vi "PH_BlackBox.set modified data.vi"(0 "i ref in":refnum<vi>, 2 "i attribute":T1={"BB Remote Controlled?"=FALSE, "GUI Refs"={"MOVE IN"=refnum, "MOVE"=refnum, "IN"=refnum, "OUT"=refnum, "REMOTE"=refnum, "GUI-Knob Move"=refnum, "GUI-Knob Move in"=refnum, "POWER ON"=refnum, "Delete"=refnum, "Function Textfield"=refnum}, "Position IN"=0, "Position OUT"=0, "BB Remote Controlled by other Instance?"=FALSE, "Recipient"="N/A", "Number"=0, "Caption Move"="", "Caption Out"="", "Caption In"=""} {"Position OUT" items=["no info", "off/false/out", "on/true/in", "Failure", "Alarm", "Status 1", "Status 2", "Status 3"]; "Position IN" items=["no info", "off/false/out", "on/true/in", "Failure", "Alarm", "Status 1", "Status 2", "Status 3"]}, 5 "error in (no error)":errorcluster) -> (14 "i ref out":refnum<vi>, 19 "error out":errorcluster)   [LabVIEW 2014, in "PH_BlackBox.lvlib"]
doc: "Writes the data into the attribute of an object. Then, the attribute dara are unlocked using the \"release\" method. Prior to calling THIS method, the attribute data must have been locked using the methods \"lock\" or \"get data to modify\".\n\n\nLicense Agreement for this software:\n\nCopyright (C)\nGesellschaft für Schwerionenforschung, GSI\nPlanckstr. 1\n64291 Darmstadt\nGermany\n\nContact: D.Beck@gsi.de \n\nThis program is free software; you can redistribute it and/or modify it under the terms of the GNU General Public License as published by the Free Software Foundation; either version 2 of the license, or (at your option) any later version.\n\nThis program is distributed in the hope that it will be useful, but WITHOUT ANY WARRANTY; without even the implied warranty of MERCHANTABILITY or FITNESS FOR A PARTICULAR PURPOSE. See the GNU General License for more details (http://www.gnu.org).\n\nGesellschaft für Schwerionenforschung, GSI\nPlanckstr. 1, 64291 Darmstadt, Germany\nFor all questions and ideas contact: M.Richter@gsi.de, H.Brand@gsi.de or D.Beck@gsi.de.\nLast update: 17-JUN-2004"
uses:
  PH_BlackBox.lvlib
  PH_BlackBox.i attribute.ctl
  PH_BlackBox.GUI Refs.ctl
  PH_Basics/PH_StatusHandler/PH_StatusHandler.Status.ctl
  CS_Core/CSObj/CSObj.lvlib
  PH_Basics/PH_StatusHandler/PH_StatusHandler.lvlib
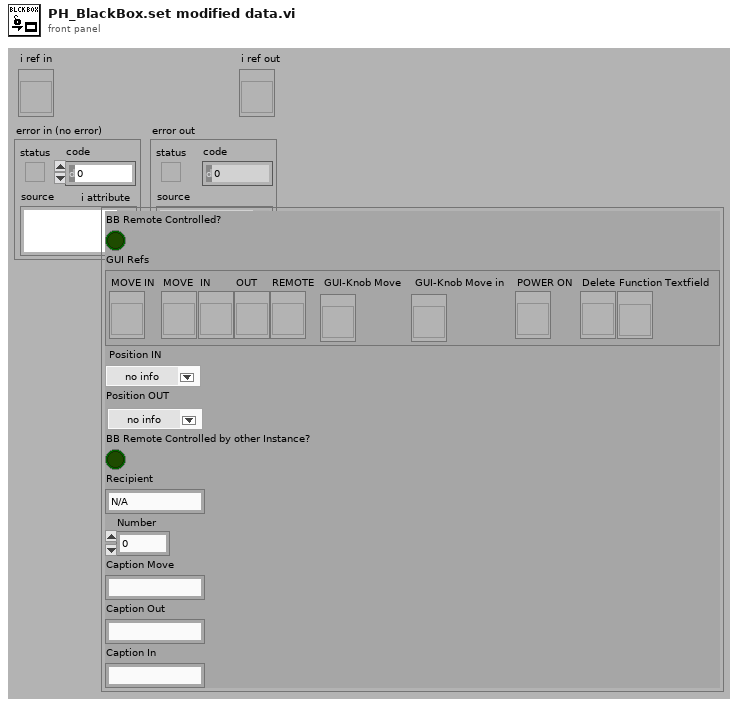
[diagram p1: front panel]
types:
  T1 = typedef "PH_BlackBox.lvlib/PH_BlackBox.i attribute.ctl" = cluster{"BB Remote Controlled?":bool, "GUI Refs":T2, "Position IN":T3, "Position OUT":T3, "BB Remote Controlled by other Instance?":bool, "Recipient":string, "Number":i32, "Caption Move":string, "Caption Out":string, "Caption In":string}
  T2 = typedef "PH_BlackBox.lvlib/PH_BlackBox.GUI Refs.ctl" = cluster{"MOVE IN":refnum<vi>, "MOVE":refnum<vi>, "IN":refnum<vi>, "OUT":refnum<vi>, "REMOTE":refnum<vi>, "GUI-Knob Move":refnum<vi>, "GUI-Knob Move in":refnum<vi>, "POWER ON":refnum<vi>, "Delete":refnum<vi>, "Function Textfield":refnum<vi>}
  T3 = typedef "PH_StatusHandler.lvlib/PH_StatusHandler.Status.ctl" = i16
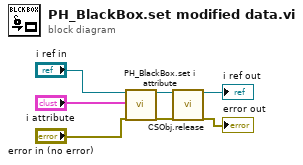
[diagram p0: block diagram]
diagram:
  n1 = call "PH_BlackBox.set i attribute.vi"("i ref in"="i ref in", "i attribute"="i attribute", "error in (no error)"="error in (no error)") -> ("i ref out"=w4:refnum<vi>, "error out"=w3:errorcluster)  [unwired: 15 in]
  n2 = call "CSObj.release.vi"("i ref in"=w4, "error in (no error)"=w3) -> ("i ref out"=→"i ref out":refnum<vi>, "error out"=→"error out":errorcluster)  [unwired: 16 in]
